vi "Record.ReverseCurrentRead.vi"(5 "Reverse Read":bool, 7 "DisableRasterFlip":bool, 10 "Line Status In":T2) -> (2 "Reverse Read":bool)   [LabVIEW 2014]
uses:
  Acquisition Engine/Acquisition Status.ctl
panel:
  # "Copyright 2014 Vidrio Technologies\nScanImage 5 software is licensed under the Apache License, Version 2.0 (the \"License\"); you may not use any files contained\nwithin the ScanImage 5 release except in compliance with the License. You may obtain a copy of the License at\n http://www.apache.org/licenses/LICENSE-2.0\nUnless required by applicable law or agreed to in writing, software distributed under the License is distributed on an\n\"AS IS\" BASIS, WITHOUT WARRANTIES OR CONDITIONS OF ANY KIND, either express or implied. See the License for the\n specific language governing permissions and limitations under the License."
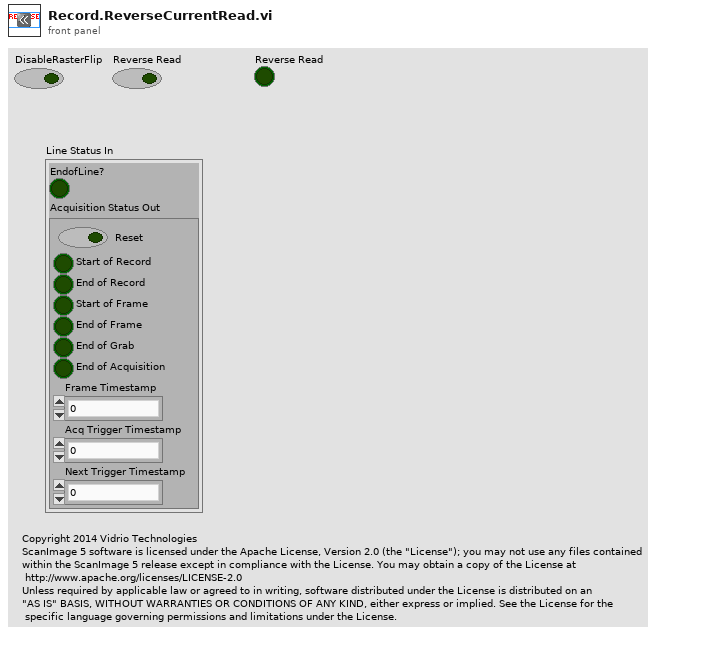
[diagram p1: front panel]
types:
  T1 = typedef "Acquisition Status.ctl" = cluster{"Reset":bool, "Start of Record":bool, "End of Record":bool, "Start of Frame":bool, "End of Frame":bool, "End of Grab":bool, "End of Acquisition":bool, "Frame Timestamp":u64, "Acq Trigger Timestamp":u64, "Next Trigger Timestamp":u64}
  T2 = cluster{"EndofLine?":bool, "Acquisition Status Out":T1}
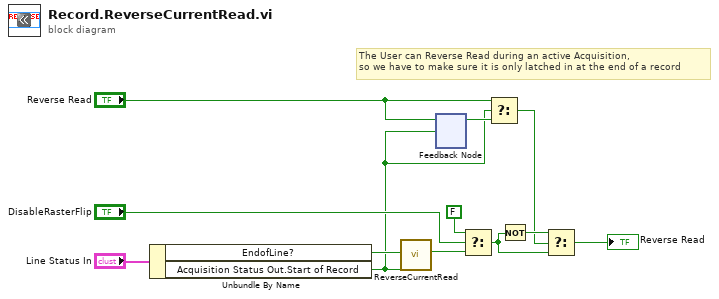
[diagram p0: block diagram]
diagram:
  # "The User can Reverse Read during an active Acquisition,\nso we have to make sure it is only latched in at the end of a record"
  n1 = Unbundle By Name("Line Status In") -> ("EndofLine?"=w12:bool, "Acquisition Status Out.Start of Record"=w2:bool)
  n2 = call "ReverseCurrentRead.vi"("Reset"=w2, "Switch Direction"=w12) -> ("Reverse Read"=w10:bool)  [unwired: 9 in]
  n3 = feedback-in #1("Reverse Read", w2) -> ()
  n4 = feedback #1() -> (w5:bool)  [unwired: 1 in]
  n5 = Select(t=FALSE, s="DisableRasterFlip", f=w10) -> (s? t:f=w7:bool)
  n6 = Select(t="Reverse Read", s=w2, f=w5) -> (s? t:f=w3:bool)
  n7 = Not(x=w7) -> (.not. x?=w8:bool)
  n8 = Select(t=w8, s=w3, f=w7) -> (s? t:f=→"Reverse Read":bool)
